vi "OpenFPGARef.vi"(1 "IP Address":string="192.168.0.21") -> (0 "FPGA VI Reference Out":T1)   [LabVIEW 2013]
uses:
  fpga-bitfile-ref.ctl
  <vilib>/userdefined/High Color/nirio_resource_hc.ctl
  <vilib>/FPGAPlugInAG/sbRIO-9602/niLvFpga_Open_sbRIO-9602.vi
  <vilib>/FPGAPlugInAG/sbRIO-9602/niLvFpga_Run_sbRIO-9602.vi
  <vilib>/rvi/interface/nirviOpenFPGA/nirviOpenFPGA.xnode
  FPGA Bitfiles/fpga-clean1_FPGATarget_FPGAMAINlock-in_FC21E42C.lvbitx
  <vilib>/rvi/interface/nirviMethod/nirviMethod.xnode
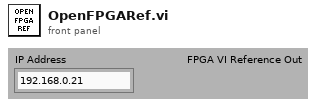
[diagram p1: front panel]
types:
  T1 = typedef "fpga-bitfile-ref.ctl" = refnum<k20>
  T2 = typedef "nirio_resource_hc.ctl" = tag
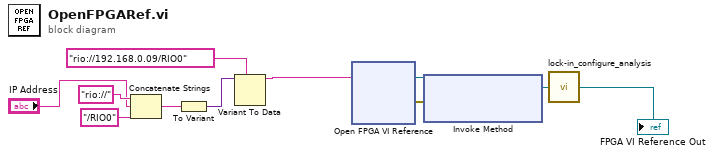
[diagram p0: block diagram]
diagram:
  n1 = Concatenate Strings("rio://" ("string"), "IP Address", "/RIO0" ("string")) -> (w11:string)
  n2 = To Variant(anything=w11) -> (Variant=w8:variant)
  n3 = Variant To Data(type=T2 "rio://192.168.0.09/RIO0" ("resource name"), Variant=w8) -> (data=w3:T2)  [unwired: 1 in, 1 out]
  n4 = xnode "Open FPGA VI Reference"("resource name"=w3) -> ("FPGA VI Reference Out"=w5:T1, "error out"=w6:errorcluster)  [unwired: 1 in]
  n5 = xnode "Invoke Method"("FPGA VI Reference In"=w5, "error in"=w6) -> ("FPGA VI Reference Out"=w4:T1)  [unwired: 1 in, 1 out]
  n6 = call "lock-in_configure_analysis.vi"("FPGA VI Reference in"=w4) -> ("FPGA VI Reference Out"=→"FPGA VI Reference Out":T1)
